vi "uTTA_GetFastSamplerate.vi"(8 "error in":errorcluster, 11 "VISA Refnum in":refnum<visa-resource-name>) -> (0 "error out":errorcluster, 1 "Fast SampleRate":i32, 3 "VISA Refnum out":refnum<visa-resource-name>, 7 "Received":string)   [LabVIEW 2021]
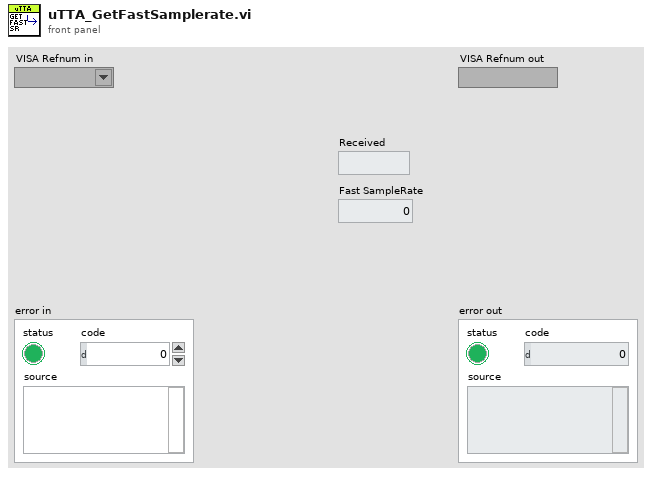
[diagram p1: front panel]
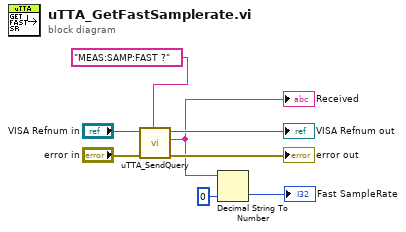
[diagram p0: block diagram]
diagram:
  n1 = call "uTTA_SendQuery.vi"("Send String"="MEAS:SAMP:FAST ?" ("format string"), "error in (no error)"="error in", "VISA Refnum in"="VISA Refnum in") -> ("error out"=→"error out":errorcluster, "Received"=w1:string, "VISA Refnum out"=→"VISA Refnum out":refnum<visa-resource-name>)  [unwired: 6 in]
  "Received" <- w1
  n2 = Decimal String To Number(string=w1, default (0L)=0 ("default value 1")) -> (number=→"Fast SampleRate":i32)  [unwired: 1 in, 1 out]
